vi "MDF4 Close File.vi"(8 "Error In":errorcluster, 11 "MDF4 File Reference in":i64) -> (0 "Error Out":errorcluster, 3 "MDF4 File Reference out":i64)   [LabVIEW 2019, in "MD4Logger Engine.lvlib"]
uses:
  MD4Logger Engine.lvlib
panel:
  out "error":i32
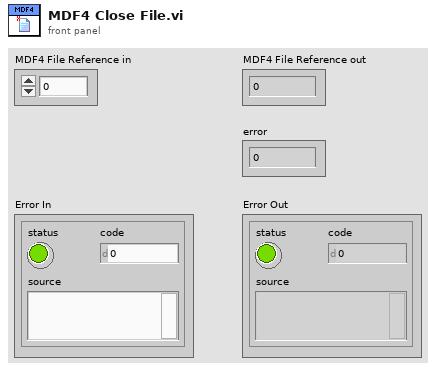
[diagram p1: front panel]
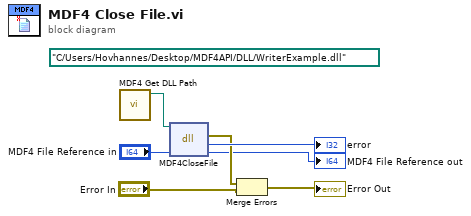
[diagram p0: block diagram]
diagram:
  (unwired) path "C:/Users/Hovhannes/Desktop/MDF4API/DLL/WriterExample.dll" ("path in")
  n1 = call "MDF4 Get DLL Path.vi"() -> ("DLL Path Out"=w1:path)  [unwired: 11 in]
  n2 = dll-call lib="C:/Users/Hovhannes/Desktop/MDF4API/DLL/WriterExample.dll" fn="MDF4CloseFile"(path in=w1, "m4"="MDF4 File Reference in") -> (error out=w5:errorcluster, "return type"=→"error":i32, "m4"=→"MDF4 File Reference out":i64)  [unwired: 2 in, 1 out]
  n3 = Merge Errors(w5, "Error In") -> (→"Error Out":errorcluster)
